vi "Open Help for Current Page.vi"(11 "Device Ref in":T1 format="%.0x") -> ()   [LabVIEW 2015]
uses:
  <vilib>/NI Veristand/Custom Device API/Custom Device Item Ref.ctl
  <vilib>/NI VeriStand/Custom Device API/Custom Device API.lvlib
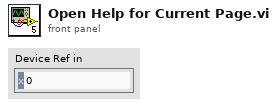
[diagram p1: front panel]
types:
  T1 = typedef "Custom Device API.lvlib/Custom Device Item Ref.ctl" = u64
  T2 = typedef "Custom Device API.lvlib/Custom Device Item Info.ctl" = cluster{"Name":string, "Is Channel":bool, "GUID":string, "Is Waveform":bool}
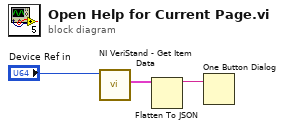
[diagram p0: block diagram]
diagram:
  n1 = call <vilib>:"NI VeriStand - Get Item Data.vi"("Item Ref in"="Device Ref in") -> ("Item Info"=w2:T2)  [unwired: 7 in, 3 out]
  n2 = Flatten To JSON(anything=w2) -> (JSON string=w1:string)  [unwired: 2 in, 1 out]
  n3 = One Button Dialog(message=w1) -> ()  [unwired: 1 in, 1 out]
